vi "Teleop_Calc_InletRange.vi"(0 "Flywheel_RPM":dbl, 7 "Dist":dbl, 11 "Use Vision?":bool) -> (8 "In Range?":bool)   [LabVIEW 2016]
panel:
  in  "upper limit":dbl
  in  "lower limit":dbl
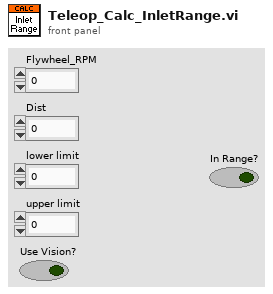
[diagram p1: front panel]
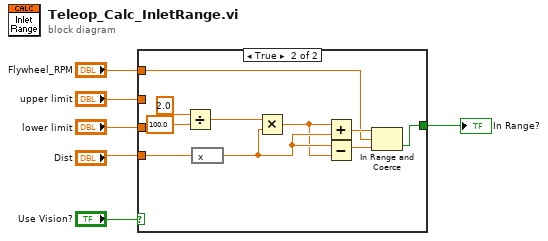
[diagram p0: block diagram]
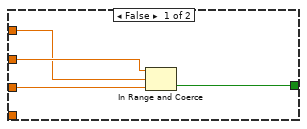
[diagram p2: hidden frame]
diagram:
  n1 = case shown="True" "Use Vision?" {
    tunnel: "Dist" -> [_ w15]
    tunnel: "lower limit" -> [w9 _]
    tunnel: "upper limit" -> [w10 _]
    tunnel: "Flywheel_RPM" -> [w8 w12]
    tunnel: [w7 w11] -> w1
    frame False {
      n2 = In Range and Coerce(upper limit=w10, x=w8, lower limit=w9) -> (In Range?=w7:bool)  [unwired: 1 out]
    }
    frame True {
      n3 = Divide(x=2.0, y=100.0) -> (x/y=w18:dbl)
      n4 = expression code="x"(w15) -> (w20:dbl)
      n5 = Multiply(x=w18, y=w20) -> (x*y=w19:dbl)
      n6 = Add(x=w19, y=w20) -> (x+y=w13:dbl)
      n7 = Subtract(x=w20, y=w19) -> (x-y=w14:dbl)
      n8 = In Range and Coerce(upper limit=w13, x=w12, lower limit=w14) -> (In Range?=w11:bool)  [unwired: 1 out]
    }
  }
  "In Range?" <- w1
